vi "Generate Random GB of Size.vi"() -> ()   [LabVIEW 2010]
uses:
  <vilib>/Utility/file.llb/Write To Spreadsheet File (string).vi
panel:
  out "GBs to Make":cluster{dbl[], dbl[], "Parameter":dbl, dbl[]}[](array[cluster])
  out "# Created":i32
  out "Grain Boundary Definition":T1={"Grain 1 Orientation"=[1.0, 0.8858401549498205, 0.0], "Grain 2 Orientation"=[1.0, 0.3745791306245927, 0.0], "Twist Angle (Deg)"=39.42112887005932, "Translation Vector"=[0.0, 0.0, 0.0]}
  out "Current Index":i32=165102
  out "Status":string="Within range!\nNow creating...\nChecking expected size\nRolling dice...\n"
  in  "Make Random GBs Tab":T2(tab)
  in  "# of Points, Translation":i32
  in  "# of Points, Angle":i32
  in  "# of Points, G2":i32
  in  "Grain 2 or Misorientation Axis":T3={"h, min"=1.0, "h, max"=1.0, "k, min"=0.0, "k, max"=1.0, "l, min"=0.0, "l, max"=1.0} caption="Grain 2 Orientation" {"h, min" format="%#_4f"; "h, max" format="%#_4f"; "k, min" format="%#_4f"; "k, max" format="%#_4f"; "l, min" format="%#_4f"; "l, max" format="%#_4f"}
  in  "Force h>k>l ?":bool=TRUE
  in  "Grain DoF Style":enum32{"Interface-Plane", "Misorientation"}(radio)
  in  "Creation Style":enum32{"Random", "Sequential"}(radio)
  in  "Grain 1 Orientation":T3={"h, min"=1.0, "h, max"=1.0, "k, min"=0.0, "k, max"=1.0, "l, min"=0.0, "l, max"=1.0} {"h, min" format="%#_4f"; "h, max" format="%#_4f"; "k, min" format="%#_4f"; "k, max" format="%#_4f"; "l, min" format="%#_4f"; "l, max" format="%#_4f"}
  in  "Angle Min":dbl caption="Twist Angle"
  in  "Angle Max":dbl=64.0 caption="Max"
  in  "Nearest Integers?":bool
  in  "Translation":T4={"T_x min"=0.0, "T_x max"=3.3, "T_y min"=0.0, "T_y max"=3.3, "T_z min"=0.0, "T_z max"=3.3} {"T_x min" format="%#_4f"; "T_x max" format="%#_4f"; "T_y min" format="%#_4f"; "T_y max" format="%#_4f"; "T_z min" format="%#_4f"; "T_z max" format="%#_4f"}
  in  "# of Points, G1":i32
  out "# of total points":i32
  in  "Max # of Atoms":i32=500
  in  "Require STEM Viewable?":bool
  in  "Collision Removal":T5={"Min Seperation Distance (A)"=2.0, "Edge Duplication Range (A)"=3.0}
  in  "Number of integers to search":i32=15
  in  "Co-incident Tolerance":dbl=0.05
  in  "Grain Growth and Geometry":T6={"Min Grain Length (A)"=10.0, "Min Angle from GB plane"=15.0, "GB Overlap Length (A)"=0.0}
  out "Expected # of atoms":i32=472
  out "# of atoms":i32=2541
  in  "Output Directory":path=path "D:/Ab-initio/GB Genie Output"
  out "Last Creation Time":T7={"Time to create primitives"=1, "Time to Grow to Box"=5932, "Time to find subset"=6894, "Time to Cleanup"=0}
  out "Structures / Minute":dbl
  in  "Stop Making GBs":bool
  in  "Start Making GBs":bool
  in  "Making GBs":bool
  in  "Conventional Unit Cell":T8={"Structure Name"="CdTe", "Lattice vector a"=[6.615785553057252, 0.0, 0.0], "Lattice vector b"=[0.0, 6.615785553057252, 0.0], "Lattice vector c"=[0.0, 0.0, 6.615785553057252], "Atoms Array"=[{"Atom Name"="Cd", "Positions (Direct)"=[[0.0, 0.0, 0.0], [0.0, 0.5, 0.5], [0.5, 0.0, 0.5], [0.5, 0.5, 0.0]], "Positions (Cartesian)"=[[0.0, 0.0, 0.0], [0.0, 3.307892776528626, 3.307892776528626], [3.307892776528626, 0.0, 3.307892776528626], [3.307892776528626, 3.307892776528626, 0.0]]}, {"Atom Name"="Te", "Positions (Direct)"=[[0.25, 0.25, 0.25], [0.75, 0.75, 0.25], [0.75, 0.25, 0.75], [0.25, 0.75, 0.75]], "Positions (Cartesian)"=[[1.653946388264313, 1.653946388264313, 1.653946388264313], [4.96183916479294, 4.96183916479294, 1.653946388264313], [4.96183916479294, 1.653946388264313, 4.96183916479294], [1.653946388264313, 4.96183916479294, 4.96183916479294]]}], "# of atoms"=8}
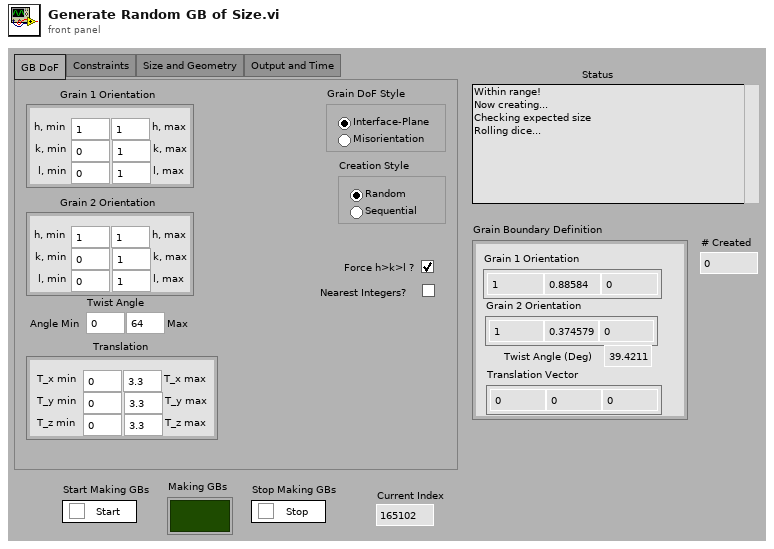
[diagram p1: front panel]
types:
  T1 = cluster{"Grain 1 Orientation":dbl[], "Grain 2 Orientation":dbl[], "Twist Angle (Deg)":dbl, "Translation Vector":dbl[]}
  T2 = enum32{"GB DoF", "Constraints", "Size and Geometry", "Output and Time"}
  T3 = cluster{"h, min":dbl, "h, max":dbl, "k, min":dbl, "k, max":dbl, "l, min":dbl, "l, max":dbl}
  T4 = cluster{"T_x min":dbl, "T_x max":dbl, "T_y min":dbl, "T_y max":dbl, "T_z min":dbl, "T_z max":dbl}
  T5 = cluster{"Min Seperation Distance (A)":dbl, "Edge Duplication Range (A)":dbl}
  T6 = cluster{"Min Grain Length (A)":dbl, "Min Angle from GB plane":dbl, "GB Overlap Length (A)":dbl}
  T7 = cluster{"Time to create primitives":u32, "Time to Grow to Box":u32, "Time to find subset":u32, "Time to Cleanup":u32}
  T8 = cluster{"Structure Name":string, "Lattice vector a":dbl[], "Lattice vector b":dbl[], "Lattice vector c":dbl[], "Atoms Array":cluster{"Atom Name":string, "Positions (Direct)":dbl[][], "Positions (Cartesian)":dbl[][]}[], "# of atoms":i32}
  T9 = cluster{dbl[], "Grain 2 Orientation":dbl[], "Twist Angle (Deg)":dbl, dbl[]}
  T10 = cluster{dbl[], "Grain 2 Orientation":dbl[], "Twist Angle (Deg)":dbl}
  T11 = typedef "NI_Matrix.lvlib/RealMatrix.ctl" = dbl[][]
  T12 = cluster{"Misorientation Angle":dbl, "Misorientation Axis, o":dbl[], "Misorientation Matrix":T11}
  T13 = cluster{"h, min":dbl, "h, max":dbl, "# of Points, G1":i32}
  T14 = cluster{"k, min":dbl, "k, max":dbl, "# of Points, G1":i32}
  T15 = cluster{"l, min":dbl, "l, max":dbl, "# of Points, G1":i32}
  T16 = cluster{"h, min":dbl, "h, max":dbl, "# of Points, G2":i32}
  T17 = cluster{"k, min":dbl, "k, max":dbl, "# of Points, G2":i32}
  T18 = cluster{"l, min":dbl, "l, max":dbl, "# of Points, G2":i32}
  T19 = cluster{"Angle Min":dbl, "Angle Max":dbl, "# of Points, Angle":i32}
  T20 = cluster{"T_x min":dbl, "T_x max":dbl, "# of Points, Translation":i32}
  T21 = cluster{"T_y min":dbl, "T_y max":dbl, "# of Points, Translation":i32}
  T22 = cluster{"T_z min":dbl, "T_z max":dbl, "# of Points, Translation":i32}
  T23 = cluster{"T_z min":dbl, "T_z max":dbl, "# of Points, Translation":i32}[]
  T24 = cluster{"T_z min":dbl, "T_z max":dbl, "# of Points, Translation":i32, "Style":enum16{"Linear Step", "Linear Pts", "Log Pts"}, string}
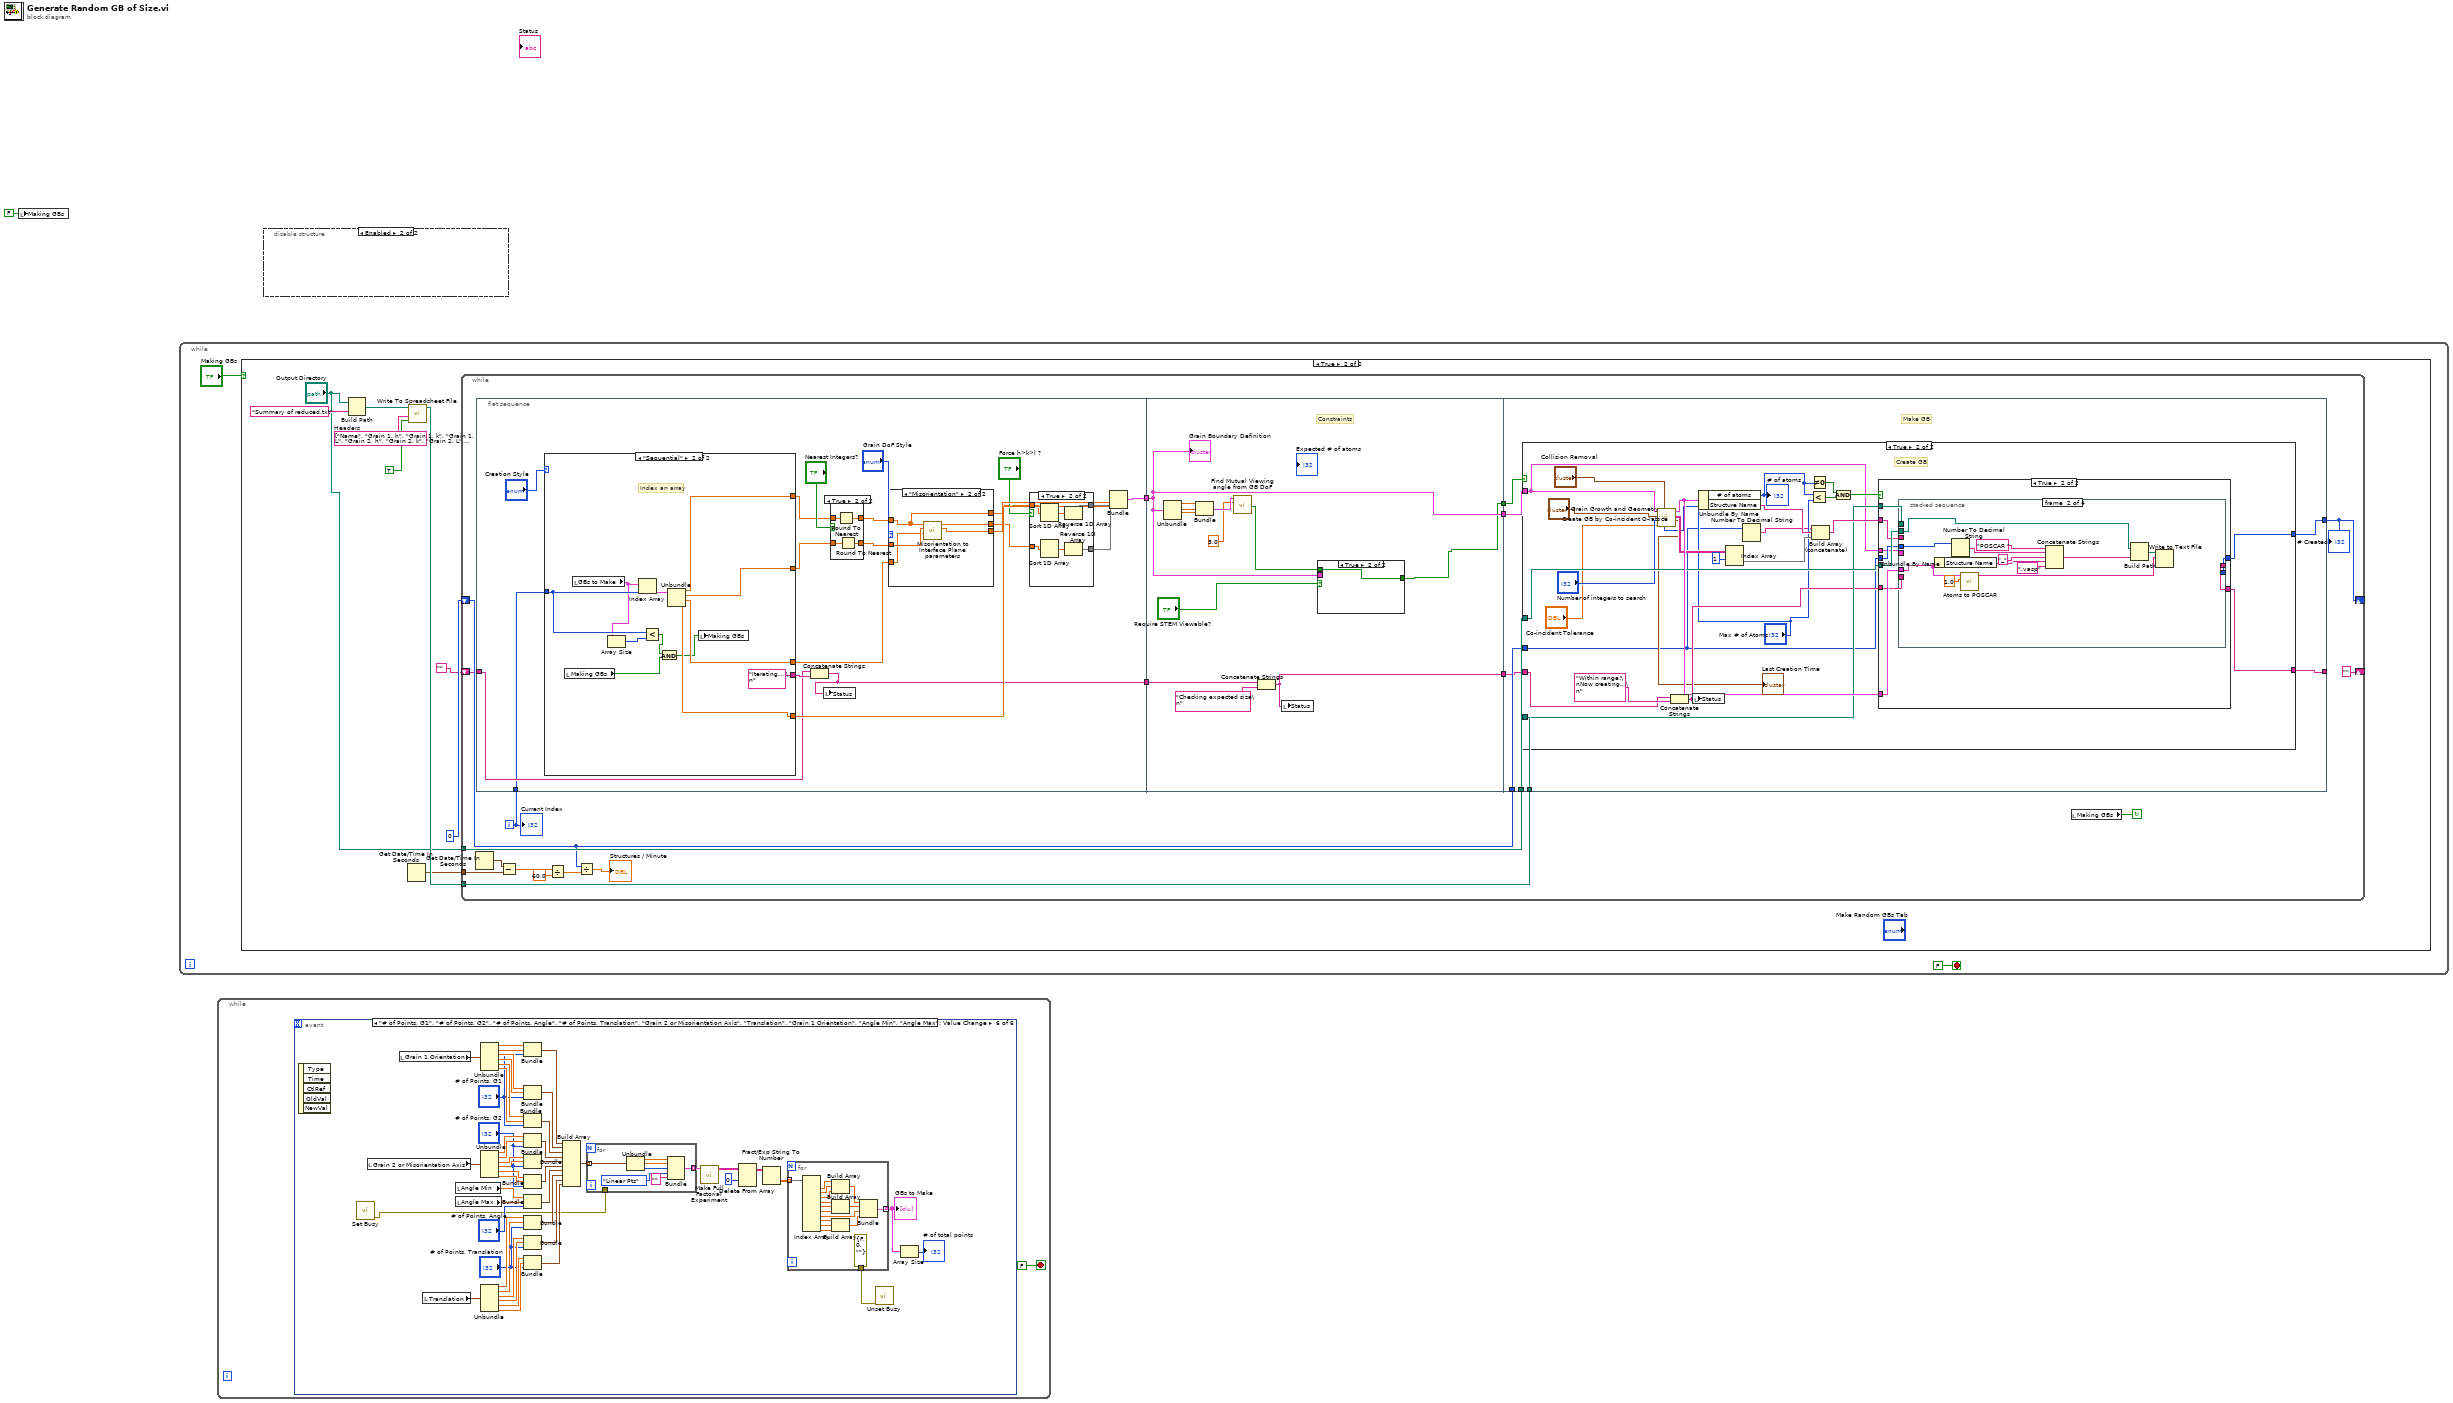
[diagram p0: block diagram]
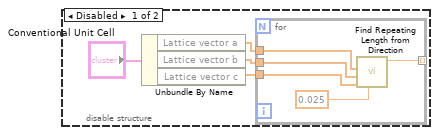
[diagram p2: hidden frame]
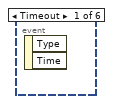
[diagram p3: hidden frame]
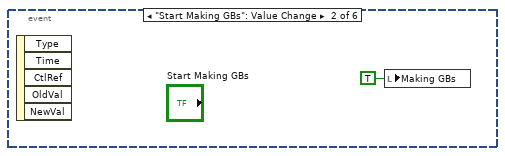
[diagram p4: hidden frame]
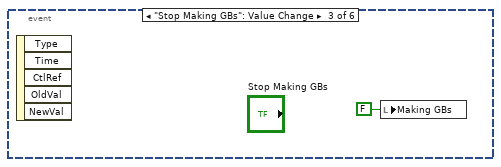
[diagram p5: hidden frame]
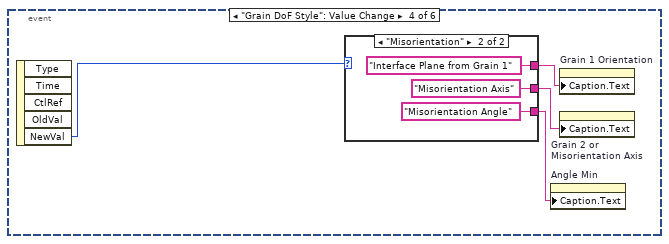
[diagram p6: hidden frame]
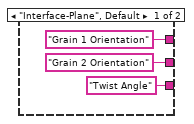
[diagram p7: hidden frame]
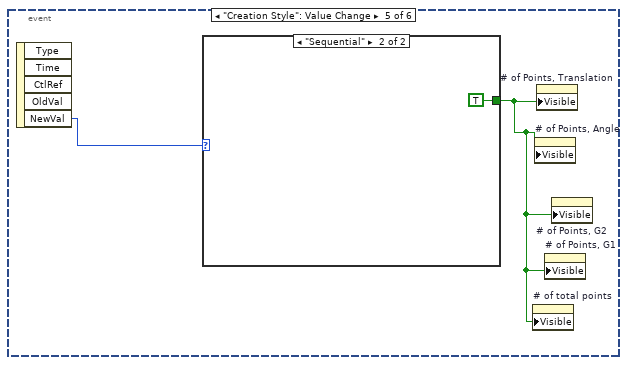
[diagram p8: hidden frame]
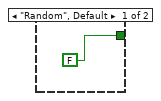
[diagram p9: hidden frame]
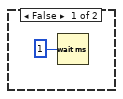
[diagram p10: hidden frame]
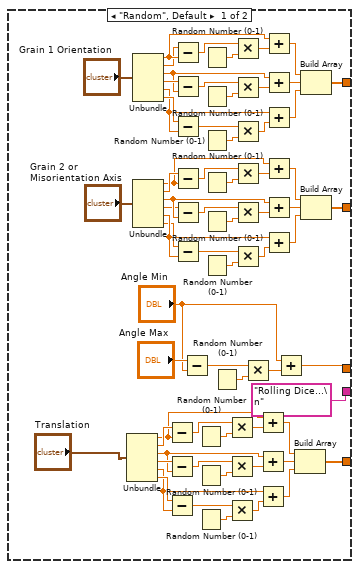
[diagram p14: hidden frame]
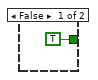
[diagram p15: hidden frame]
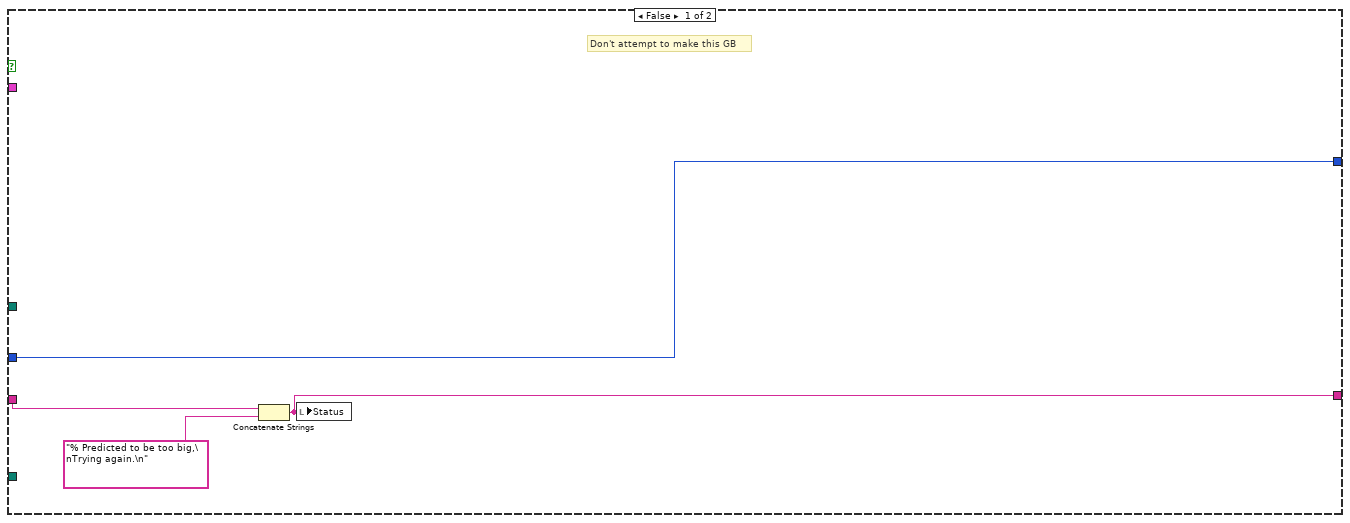
[diagram p16: hidden frame]
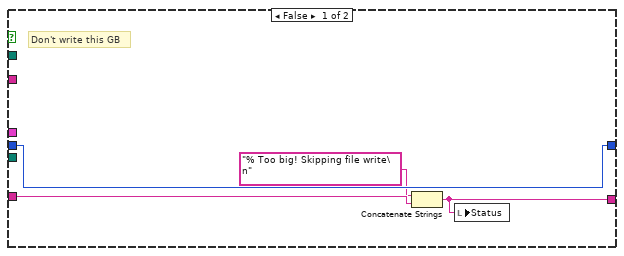
[diagram p17: hidden frame]
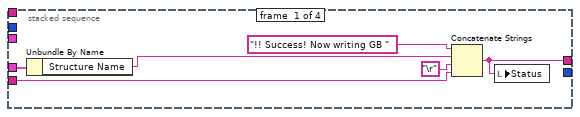
[diagram p18: hidden frame]
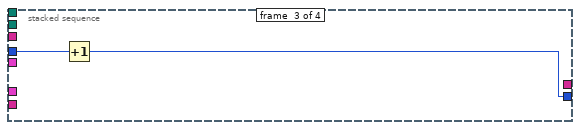
[diagram p19: hidden frame]
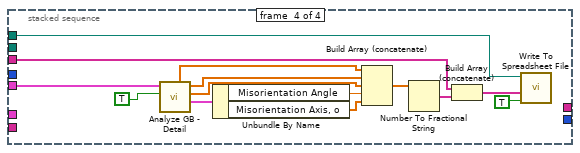
[diagram p20: hidden frame]
diagram:
  n1 = local write "Making GBs"(FALSE ("Making GBs")) -> ()
  n2 = while {
    stop <- FALSE stop-if-true
    n3 = case shown="True" "Making GBs" {
      frame False {
        n4 = Wait (ms)(milliseconds to wait=u32 1) -> ()  [unwired: 1 out]
      }
      frame True {
        w10 = string[] ["Name", "Grain 1, h", "Grain 1, k", "Grain 1, L", "Grain 2, h", "Grain 2, k", "Grain 2, L", "Twist Angle (Deg)", "Translation Tx", "Translation Ty", "Translation Tz", "Tilt Angle (Deg)", "Viewing Angle, h", "Viewing Angle, k", "Viewing Angle, L", "Grain 1 Length (factor)", "Grain 2 Length (factor", "Max Grain Height (A)", "Max Grain Width (A)", "Grain 1 Start", "Overlap Region (A)", "Reduction Slab X", "Reduction Slab Y", "Reduction Tolerance (A)", "Min Atomic Separation Distance", "Edge Duplication Range", "# of Atoms", "STEM Direction,h", "STEM Direction,k", "STEM Direction,l", "Grain 1, [h]", "Grain 1, [k]", "Grain 1, [L]", "Grain 2, [h]", "Grain 2, [k]", "Grain 2, [L]", "Misorientaton Angle (Deg)", "Misorientation Axis, h", "Misorientation Axis, k", "Misorientation Axis, l"]  # Headers
        n5 = Build Path(base path="Output Directory", name or relative path="Summary of reduced.txt") -> (appended path=w11:path)
        n6 = Get Date/Time In Seconds() -> (seconds since 1Jan1904=w6:timestamp)
        n7 = call-poly <vilib>:"Write To Spreadsheet File.vi"("append to file? (new file:F)"=TRUE, "1D data"=w10, "file path (dialog if empty)"=w11) -> ("new file path (Not A Path if cancelled)"=w8:path)  [unwired: 5 in]
        n8 = while {
          shift-right: [w22] -> _
          shift-left: 0 -> [w23]
          tunnel: w6 -> [w29]
          tunnel: "Output Directory" -> [w25]
          tunnel: w8 -> [w24]
          shift-right: [""] -> _
          shift-left: "" -> [w21]
          i -> [w14]
          stop <- w19 continue-if-true
          n9 = Get Date/Time In Seconds() -> (seconds since 1Jan1904=w17:timestamp)
          n10 = flat-sequence {
            tunnel: w21 -> [w34]
            tunnel: [w37] -> w16
            tunnel: [w35] -> w15
            tunnel: w14 -> [w33]
            tunnel: [w162] -> w27
            tunnel: [w154] -> w26
            tunnel: [w164] -> w20
            tunnel: w16 -> [w162]
            tunnel: w15 -> [w157]
            tunnel: w27 -> [w171]
            tunnel: w26 -> [w175]
            tunnel: w25 -> [w174]
            tunnel: w24 -> [w173]
            tunnel: w23 -> [w172]
            tunnel: [w170] -> w22
            tunnel: w20 -> [w169]
            tunnel: [w168] -> _
            frame #0 {
              n11 = case shown="\"Sequential\"" "Creation Style" {
                tunnel: [w104 w151] -> w39
                tunnel: [w103 w150] -> w40
                tunnel: [w97 w149] -> w45
                tunnel: [w78 w148] -> w52
                tunnel: ["Rolling Dice...\n" ("string") "Iterating... \n" ("string")] -> w36
                tunnel: w33 -> [_ w147]
                frame "Random", Default {
                  n12 = Unbundle("Translation") -> ("T_x min"=w76:dbl, "T_x max"=w80:dbl, "T_y min"=w87:dbl, "T_y max"=w88:dbl, "T_z min"=w89:dbl, "T_z max"=w90:dbl)
                  n13 = Unbundle("Grain 1 Orientation") -> ("h, min"=w130:dbl, "h, max"=w127:dbl, "k, min"=w135:dbl, "k, max"=w136:dbl, "l, min"=w137:dbl, "l, max"=w138:dbl)
                  n14 = Unbundle("Grain 2 or Misorientation Axis") -> ("h, min"=w77:dbl, "h, max"=w125:dbl, "k, min"=w118:dbl, "k, max"=w117:dbl, "l, min"=w116:dbl, "l, max"=w115:dbl)
                  n15 = Subtract(x=w80, y=w76) -> (x-y=w81:dbl)
                  n16 = Subtract(x=w88, y=w87) -> (x-y=w84:dbl)
                  n17 = Subtract(x=w90, y=w89) -> (x-y=w85:dbl)
                  n18 = Subtract(x=w127, y=w130) -> (x-y=w128:dbl)
                  n19 = Subtract(x=w136, y=w135) -> (x-y=w132:dbl)
                  n20 = Subtract(x=w138, y=w137) -> (x-y=w133:dbl)
                  n21 = Subtract(x=w125, y=w77) -> (x-y=w124:dbl)
                  n22 = Subtract(x=w117, y=w118) -> (x-y=w121:dbl)
                  n23 = Subtract(x=w115, y=w116) -> (x-y=w120:dbl)
                  n24 = Subtract(x="Angle Max", y="Angle Min") -> (x-y=w100:dbl)
                  n25 = Random Number (0-1)() -> (number: 0 to 1=w91:dbl)
                  n26 = Random Number (0-1)() -> (number: 0 to 1=w92:dbl)
                  n27 = Random Number (0-1)() -> (number: 0 to 1=w93:dbl)
                  n28 = Random Number (0-1)() -> (number: 0 to 1=w139:dbl)
                  n29 = Random Number (0-1)() -> (number: 0 to 1=w140:dbl)
                  n30 = Random Number (0-1)() -> (number: 0 to 1=w141:dbl)
                  n31 = Random Number (0-1)() -> (number: 0 to 1=w114:dbl)
                  n32 = Random Number (0-1)() -> (number: 0 to 1=w113:dbl)
                  n33 = Random Number (0-1)() -> (number: 0 to 1=w112:dbl)
                  n34 = Random Number (0-1)() -> (number: 0 to 1=w102:dbl)
                  n35 = Multiply(x=w81, y=w91) -> (x*y=w82:dbl)
                  n36 = Multiply(x=w84, y=w92) -> (x*y=w83:dbl)
                  n37 = Multiply(x=w85, y=w93) -> (x*y=w86:dbl)
                  n38 = Multiply(x=w128, y=w139) -> (x*y=w129:dbl)
                  n39 = Multiply(x=w132, y=w140) -> (x*y=w131:dbl)
                  n40 = Multiply(x=w133, y=w141) -> (x*y=w134:dbl)
                  n41 = Multiply(x=w124, y=w114) -> (x*y=w123:dbl)
                  n42 = Multiply(x=w121, y=w113) -> (x*y=w122:dbl)
                  n43 = Multiply(x=w120, y=w112) -> (x*y=w119:dbl)
                  n44 = Multiply(x=w100, y=w102) -> (x*y=w101:dbl)
                  n45 = Add(x=w76, y=w82) -> (x+y=w94:dbl)
                  n46 = Add(x=w87, y=w83) -> (x+y=w95:dbl)
                  n47 = Add(x=w89, y=w86) -> (x+y=w96:dbl)
                  n48 = Add(x=w130, y=w129) -> (x+y=w110:dbl)
                  n49 = Add(x=w135, y=w131) -> (x+y=w109:dbl)
                  n50 = Add(x=w137, y=w134) -> (x+y=w108:dbl)
                  n51 = Add(x=w77, y=w123) -> (x+y=w107:dbl)
                  n52 = Add(x=w118, y=w122) -> (x+y=w106:dbl)
                  n53 = Add(x=w116, y=w119) -> (x+y=w105:dbl)
                  n54 = Add(x="Angle Min", y=w101) -> (x+y=w97:dbl)
                  n55 = Build Array(w94, w95, w96) -> (w78:dbl[])
                  n56 = Build Array(w110, w109, w108) -> (w104:dbl[])
                  n57 = Build Array(w107, w106, w105) -> (w103:dbl[])
                }
                frame "Sequential" {
                  # "Index an array"
                  n58 = local read "Making GBs"() -> (w143:bool)
                  n59 = local read "GBs to Make"() -> (w146:cluster{dbl[], dbl[], "Parameter":dbl, dbl[]}[])
                  n60 = Array Size(array=w146) -> (size(s)=w145:i32)
                  n61 = Index Array(array=w146, index=w147) -> (element=w152:cluster{dbl[], dbl[], "Parameter":dbl, dbl[]})
                  n62 = Less?(x=w147, y=w145) -> (x < y?=w144:bool)
                  n63 = And(x=w144, y=w143) -> (x .and. y?=w142:bool)
                  n64 = Unbundle(w152) -> (w151:dbl[], w150:dbl[], "Parameter"=w149:dbl, w148:dbl[])
                  n65 = local write "Making GBs"(w142) -> ()
                }
              }
              n66 = Concatenate Strings(w34, w36) -> (w35:string)
              n67 = local write "Status"(w35) -> ()
              n68 = case shown="True" "Nearest Integers?" {
                tunnel: [w69 w74] -> w44
                tunnel: [w70 w73] -> w43
                tunnel: w39 -> [w70 w72]
                tunnel: w40 -> [w69 w71]
                frame False {
                }
                frame True {
                  n69 = Round To Nearest(number=w72) -> (nearest integer value=w73:dbl[])
                  n70 = Round To Nearest(number=w71) -> (nearest integer value=w74:dbl[])
                }
              }
              n71 = case shown="\"Misorientation\"" "Grain DoF Style" {
                tunnel: w43 -> [w63 w65]
                tunnel: w44 -> [w62 w68]
                tunnel: w45 -> [w61 w67]
                tunnel: [w62 w66] -> w48
                tunnel: [w63 w65] -> w46
                tunnel: [w61 w64] -> w51
                frame "Interface-Plane", Default {
                }
                frame "Misorientation" {
                  n72 = call "Misorientation to Interface Plane parameters.vi"("Misorientation Angle"=w67, "Misorientation Axis, o"=w68, "Grain 1 Orientation"=w65) -> ("Twist Angle (Deg)"=w64:dbl, "Grain 2 Orientation"=w66:dbl[])  [unwired: 5 in, 2 out]
                }
              }
              n73 = case shown="True" "Force h>k>l ?" {
                tunnel: [w54 w58] -> w49
                tunnel: w46 -> [w54 w60]
                tunnel: w48 -> [w53 w56]
                tunnel: [w53 w55] -> w50
                frame False {
                }
                frame True {
                  n74 = Sort 1D Array(array=w60) -> (sorted array=w59:dbl[])
                  n75 = Sort 1D Array(array=w56) -> (sorted array=w57:dbl[])
                  n76 = Reverse 1D Array(array=w59) -> (reversed array=w58:dbl[])
                  n77 = Reverse 1D Array(array=w57) -> (reversed array=w55:dbl[])
                }
              }
              n78 = Bundle(w49, "Grain 2 Orientation"=w50, "Twist Angle (Deg)"=w51, w52) -> (w37:T9)  [unwired: 1 in]
            }
            frame #1 {
              # "Constraints"
              n79 = Unbundle(w162) -> (w161:dbl[], "Grain 2 Orientation"=w160:dbl[], "Twist Angle (Deg)"=w159:dbl)  [unwired: 1 out]
              n80 = Bundle(w161, "Grain 2 Orientation"=w160, "Twist Angle (Deg)"=w159) -> (w158:T10)  [unwired: 1 in]
              n81 = call "Find Mutual Viewing angle from GB DoF.vi"("Viewing Angle Tolerance (Deg)"=3.0 ("Integer Tolerance"), "Grain Boundary Macro DoF"=w158) -> ("STEM Viewable?"=w155:bool)  [unwired: 7 in, 2 out]
              n82 = Concatenate Strings(w157, "Checking expected size\n" ("string")) -> (w164:string)
              n83 = local write "Status"(w164) -> ()
              n84 = case shown="True" "Require STEM Viewable?" {
                tunnel: w162 -> [_ _]
                tunnel: [TRUE ("STEM Viewable?") w167] -> w154
                tunnel: w155 -> [_ w167]
                frame False {
                }
                frame True {
                }
              }
              "Grain Boundary Definition" <- w162
            }
            frame #2 {
              # "Make GB"
              n85 = case shown="True" w175 {
                tunnel: w174 -> [_ w199]
                tunnel: w173 -> [_ w198]
                tunnel: w172 -> [w179 w181]
                tunnel: w171 -> [_ w188]
                tunnel: [w179 w193] -> w170
                tunnel: w169 -> [w178 w191]
                tunnel: [w176 w189] -> w168
                frame False {
                  # "Don't attempt to make this GB"
                  n86 = Concatenate Strings(w178, "% Predicted to be too big,\nTrying again.\n" ("string")) -> (w176:string)
                  n87 = local write "Status"(w176) -> ()
                }
                frame True {
                  # "Create GB"
                  n88 = call "Create GB by Co-incident O-lattice.vi"("Max # of atoms"="Max # of Atoms", "Collision Removal"="Collision Removal", "Co-incident Tolerance"="Co-incident Tolerance", "Number of integers to search"="Number of integers to search", "Grain Growth and Geometry"="Grain Growth and Geometry", "Grain Boundary Definition"=w188) -> ("Creation Time"=→"Last Creation Time":T7, "GB Data"=w200:string[][], "Grain Boundary"=w201:T8)  [unwired: 3 in]
                  n89 = Concatenate Strings(w191, "Within range!\nNow creating...\n" ("string")) -> (w190:string)
                  n90 = local write "Status"(w190) -> ()
                  n91 = Unbundle By Name(w201) -> ("# of atoms"=w197:i32, "Structure Name"=w205:string)
                  "# of atoms" <- w197
                  n92 = Index Array(array=w200, index (row)=1) -> (element=w203:string[])  [unwired: 1 in]
                  n93 = Number To Decimal String(number=w181) -> (decimal integer string=w180:string)  [unwired: 1 in]
                  n94 = Less?(x=w197, y="Max # of Atoms") -> (x < y?=w195:bool)
                  n95 = Not Equal To 0?(x=w197) -> (x != 0?=w196:bool)
                  n96 = Build Array (concatenate)(w180, w205, w203) -> (w204:string[])
                  n97 = Compound Arithmetic op=AND(w196, w195) -> (w194:bool)
                  n98 = case shown="True" w194 {
                    tunnel: w181 -> [w209 w216]
                    tunnel: [w209 w215] -> w193
                    tunnel: w201 -> [_ w218]
                    tunnel: w204 -> [_ w213]
                    tunnel: w199 -> [_ w217]
                    tunnel: w198 -> [_ w214]
                    tunnel: w190 -> [w208 w211]
                    tunnel: [w207 w210] -> w189
                    tunnel: w188 -> [_ w212]
                    frame False {
                      # "Don't write this GB"
                      n99 = Concatenate Strings("% Too big! Skipping file write\n" ("string"), w208) -> (w207:string)
                      n100 = local write "Status"(w207) -> ()
                    }
                    frame True {
                      n101 = stacked-sequence {
                        tunnel: w218 -> [w222 w225 _ _]
                        tunnel: w217 -> [_ w226 _ _]
                        tunnel: w216 -> [_ w232 w238 _]
                        tunnel: [_ _ w237 _] -> w215
                        tunnel: w214 -> [_ _ _ w252]
                        tunnel: w213 -> [_ _ _ w250]
                        tunnel: w212 -> [_ _ _ w244]
                        tunnel: w211 -> [w220 _ _ _]
                        tunnel: [w219 _ _ _] -> w210
                        frame #0 {
                          n102 = Unbundle By Name(w222) -> ("Structure Name"=w221:string)
                          n103 = Concatenate Strings("!! Success! Now writing GB " ("string"), w221, "\r", w220) -> (w219:string)
                          n104 = local write "Status"(w219) -> ()
                        }
                        frame #1 {
                          n105 = Unbundle By Name(w225) -> ("Structure Name"=w229:string)
                          n106 = Number To Decimal String(number=w232) -> (decimal integer string=w236:string)  [unwired: 1 in]
                          n107 = call "Atoms to POSCAR.vi"("Volume Factor"=1.0, "Atomic Structure"=w225) -> ("POSCAR File"=w231:string)  [unwired: 9 in]
                          n108 = Concatenate Strings("POSCAR " ("string"), w236, "_" ("string"), w229, ".vasp" ("string")) -> (w235:string)
                          n109 = Build Path(base path=w226, name or relative path=w235) -> (appended path=w227:path)
                          n110 = Write to Text File(file (use dialog)=w227, text=w231) -> ()  [unwired: 2 in, 3 out]
                        }
                        frame #2 {
                          n111 = Increment(x=w238) -> (x+1=w237:i32)
                        }
                        frame #3 {
                          n112 = call "Analyze GB - Detail.vi"("Find Integer Rep?"=TRUE, "Grain Boundary Definition"=w244) -> ("Misorientation"=w248:T12, "Grain 2 Integers"=w247:dbl[], "Grain 1 Integers"=w246:dbl[], "Suggested view direction"=w239:dbl[])  [unwired: 2 in, 4 out]
                          n113 = Unbundle By Name(w248) -> ("Misorientation Angle"=w243:dbl, "Misorientation Axis, o"=w242:dbl[])
                          n114 = Build Array (concatenate)(w239, w246, w247, w243, w242) -> (w241:dbl[])
                          n115 = Number To Fractional String(number=w241) -> (F-format string=w240:string[])  [unwired: 3 in]
                          n116 = Build Array (concatenate)(w250, w240) -> (w249:string[])
                          n117 = call-poly <vilib>:"Write To Spreadsheet File.vi"("append to file? (new file:F)"=TRUE, "1D data"=w249, "file path (dialog if empty)"=w252) -> ()  [unwired: 5 in, 1 out]
                        }
                      }
                    }
                  }
                }
              }
            }
          }
          n118 = Subtract(x=w17, y=w29) -> (x-y=w31:dbl)
          n119 = Divide(x=w31, y=60.0) -> (x/y=w28:dbl)
          n120 = Divide(x=w23, y=w28) -> (x/y=→"Structures / Minute":dbl)
          n121 = local read "Making GBs"() -> (w19:bool)
          "Current Index" <- w14
          "# Created" <- w22
        }
      }
    }
  }
  n122 = while {
    stop <- FALSE stop-if-true
    n123 = event shown="[5] \"# of Points, G1\", \"# of Points, G2\", \"# of Points, Angle\", \"# of Points, Translation\", \"Grain 2 or Misorientation Axis\", \"Translation\", \"Grain 1 Orientation\", \"Angle Min\", \"Angle Max\": Value Change" {
      selector: _ -> [_ _ _ _ _ _]
      dyn-events: _ -> [_ _ _ _ _ _]
      timeout: _ -> [_ _ _ _ _ _]
      event Timeout {
        n124 = event-data() -> ()  [unwired: 1 in, 2 out]
      }
      event "Start Making GBs": Value Change {
        n125 = event-data() -> ()  [unwired: 1 in, 5 out]
        n126 = local write "Making GBs"(TRUE ("Making GBs")) -> ()
      }
      event "Stop Making GBs": Value Change {
        n127 = event-data() -> ()  [unwired: 1 in, 5 out]
        n128 = local write "Making GBs"(FALSE ("Making GBs")) -> ()
      }
      event "Grain DoF Style": Value Change {
        n129 = event-data() -> ("NewVal"=w259:enum32{"Interface-Plane", "Misorientation"})  [unwired: 1 in, 4 out]
        n130 = case shown="\"Misorientation\"" w259 {
          tunnel: ["Grain 1 Orientation" ("Caption.Text") "Interface Plane from Grain 1" ("Caption.Text")] -> w258
          tunnel: ["Grain 2 Orientation" ("Caption.Text") "Misorientation Axis" ("Caption.Text")] -> w257
          tunnel: ["Twist Angle" ("Caption.Text") "Misorientation Angle" ("Caption.Text")] -> w256
          frame "Interface-Plane", Default {
          }
          frame "Misorientation" {
          }
        }
        n131 = property on="Angle Min" class="DigNum (strict)"("Caption.Text"=w256) -> ()  [unwired: 2 in, 2 out]
        n132 = property on="Grain 1 Orientation" class="Clust (strict)"("Caption.Text"=w258) -> ()  [unwired: 2 in, 2 out]
        n133 = property on="Grain 2 or Misorientation Axis" class="Clust (strict)"("Caption.Text"=w257) -> ()  [unwired: 2 in, 2 out]
      }
      event "Creation Style": Value Change {
        n134 = event-data() -> ("NewVal"=w267:enum32{"Random", "Sequential"})  [unwired: 1 in, 4 out]
        n135 = case shown="\"Sequential\"" w267 {
          tunnel: [FALSE ("Visible") TRUE ("Visible")] -> w266
          frame "Random", Default {
          }
          frame "Sequential" {
          }
        }
        n136 = property on="# of total points" class="DigNum (strict)"("Visible"=w266) -> ()  [unwired: 2 in, 2 out]
        n137 = property on="# of Points, Angle" class="DigNum (strict)"("Visible"=w266) -> ()  [unwired: 2 in, 2 out]
        n138 = property on="# of Points, Translation" class="DigNum (strict)"("Visible"=w266) -> ()  [unwired: 2 in, 2 out]
        n139 = property on="# of Points, G1" class="DigNum (strict)"("Visible"=w266) -> ()  [unwired: 2 in, 2 out]
        n140 = property on="# of Points, G2" class="DigNum (strict)"("Visible"=w266) -> ()  [unwired: 2 in, 2 out]
      }
      event "# of Points, G1", "# of Points, G2", "# of Points, Angle", "# of Points, Translation", "Grain 2 or Misorientation Axis", "Translation", "Grain 1 Orientation", "Angle Min", "Angle Max": Value Change {
        n141 = event-data() -> ()  [unwired: 1 in, 5 out]
        n142 = call <vilib>:"Set Busy.vi"() -> ("error out"=w271:errorcluster)  [unwired: 10 in, 1 out]
        n143 = local read "Grain 2 or Misorientation Axis"() -> (w303:T3)
        n144 = local read "Grain 1 Orientation"() -> (w316:T3)
        n145 = local read "Translation"() -> (w294:T4)
        n146 = local read "Angle Min"() -> (w293:dbl)
        n147 = local read "Angle Max"() -> (w292:dbl)
        n148 = Unbundle(w316) -> ("h, min"=w315:dbl, "h, max"=w314:dbl, "k, min"=w313:dbl, "k, max"=w312:dbl, "l, min"=w311:dbl, "l, max"=w310:dbl)
        n149 = Unbundle(w303) -> ("h, min"=w304:dbl, "h, max"=w305:dbl, "k, min"=w306:dbl, "k, max"=w307:dbl, "l, min"=w308:dbl, "l, max"=w309:dbl)
        n150 = Unbundle(w294) -> ("T_x min"=w300:dbl, "T_x max"=w299:dbl, "T_y min"=w298:dbl, "T_y max"=w297:dbl, "T_z min"=w296:dbl, "T_z max"=w295:dbl)
        n151 = Bundle("h, min"=w315, "h, max"=w314, "# of Points, G1"="# of Points, G1") -> (w289:T13)  [unwired: 1 in]
        n152 = Bundle("k, min"=w313, "k, max"=w312, "# of Points, G1"="# of Points, G1") -> (w288:T14)  [unwired: 1 in]
        n153 = Bundle("l, min"=w311, "l, max"=w310, "# of Points, G1"="# of Points, G1") -> (w287:T15)  [unwired: 1 in]
        n154 = Bundle("h, min"=w304, "h, max"=w305, "# of Points, G2"="# of Points, G2") -> (w286:T16)  [unwired: 1 in]
        n155 = Bundle("k, min"=w306, "k, max"=w307, "# of Points, G2"="# of Points, G2") -> (w285:T17)  [unwired: 1 in]
        n156 = Bundle("l, min"=w308, "l, max"=w309, "# of Points, G2"="# of Points, G2") -> (w284:T18)  [unwired: 1 in]
        n157 = Bundle("Angle Min"=w293, "Angle Max"=w292, "# of Points, Angle"="# of Points, Angle") -> (w283:T19)  [unwired: 1 in]
        n158 = Bundle("T_x min"=w300, "T_x max"=w299, "# of Points, Translation"="# of Points, Translation") -> (w282:T20)  [unwired: 1 in]
        n159 = Bundle("T_y min"=w298, "T_y max"=w297, "# of Points, Translation"="# of Points, Translation") -> (w281:T21)  [unwired: 1 in]
        n160 = Bundle("T_z min"=w296, "T_z max"=w295, "# of Points, Translation"="# of Points, Translation") -> (w280:T22)  [unwired: 1 in]
        n161 = Build Array(w289, w288, w287, w286, w285, w284, w283, w282, w281, w280) -> (w279:T23)
        n162 = for {
          tunnel: w279 -> [w339] mode=indexing
          tunnel: [w334] -> w278 mode=indexing
          tunnel: w271 -> [_]
          n163 = Unbundle(w339) -> ("T_z min"=w338:dbl, "T_z max"=w337:dbl, "# of Points, Translation"=w336:i32)
          n164 = Bundle("T_z min"=w338, "T_z max"=w337, "# of Points, Translation"=w336, "Style"=enum16{"Linear Step", "Linear Pts", "Log Pts"}."Linear Pts", "") -> (w334:T24)  [unwired: 1 in]
        }
        n165 = call "Make Full Factorial Experiment.vi"("Array of Array Settings"=w278) -> ("Full Factorial Design"=w277:string[][])  [unwired: 10 in]
        n166 = Delete From Array(array=w277, index (row)=0) -> (array with subset deleted=w275:string[][])  [unwired: 2 in, 1 out]
        n167 = Fract/Exp String To Number(string=w275) -> (number=w274:dbl[][])  [unwired: 3 in, 1 out]
        n168 = for {
          tunnel: w274 -> [w332] mode=indexing
          tunnel: [w318] -> w273 mode=indexing
          tunnel: [errorcluster {"status"=FALSE, "code"=0, "source"=""} ("error in (no error)")] -> w270
          n169 = Index Array(array=w332) -> (element #1=w331:dbl, element #2=w330:dbl, element #3=w329:dbl, element #4=w328:dbl, element #5=w327:dbl, element #6=w326:dbl, element #7=w320:dbl, element #8=w325:dbl, element #9=w324:dbl, element #10=w323:dbl)  [unwired: 10 in]
          n170 = Build Array(w331, w330, w329) -> (w322:dbl[])
          n171 = Build Array(w328, w327, w326) -> (w321:dbl[])
          n172 = Build Array(w325, w324, w323) -> (w319:dbl[])
          n173 = Bundle(w322, w321, "Parameter"=w320, w319) -> (w318:cluster{dbl[], dbl[], "Parameter":dbl, dbl[]})  [unwired: 1 in]
        }
        "GBs to Make" <- w273
        n174 = call <vilib>:"Unset Busy.vi"("error in (no error)"=w270) -> ()  [unwired: 10 in, 1 out]
        n175 = Array Size(array=w273) -> (size(s)=→"# of total points":i32)
      }
    }
  }
  n176 = disable-structure shown="Enabled" {
    frame Disabled {
      n177 = Unbundle By Name("Conventional Unit Cell") -> ("Lattice vector a"=w341:dbl[], "Lattice vector b"=w342:dbl[], "Lattice vector c"=w343:dbl[])
      n178 = for {
        tunnel: w341 -> [w348]
        tunnel: w342 -> [w347]
        tunnel: w343 -> [w346]
        tunnel: [w344] -> _ mode=indexing
        n179 = call "Find Repeating Length from Direction.vi"("Tolerance"=0.025, "Lattice vector c"=w346, "Lattice vector b"=w347, "Lattice vector a"=w348) -> ("Repeating Length (A)"=w344:dbl)  [unwired: 7 in]
      }
    }
    frame Enabled {
    }
  }
